vi "__Destroy.vi"(8 "error in (no error)":errorcluster, 11 "ClashRoyale in":refnum<class "ClashRoyale.lvclass">) -> (0 "error out":errorcluster)   [LabVIEW 2020, in "ClashRoyale.lvclass"]
uses:
  ClashRoyale.lvclass
  ClashRoyale.lvclass/ClashRoyale.ctl
  <vilib>/drjdpowell/SQLite Library/SQL Connection/Connection.lvclass
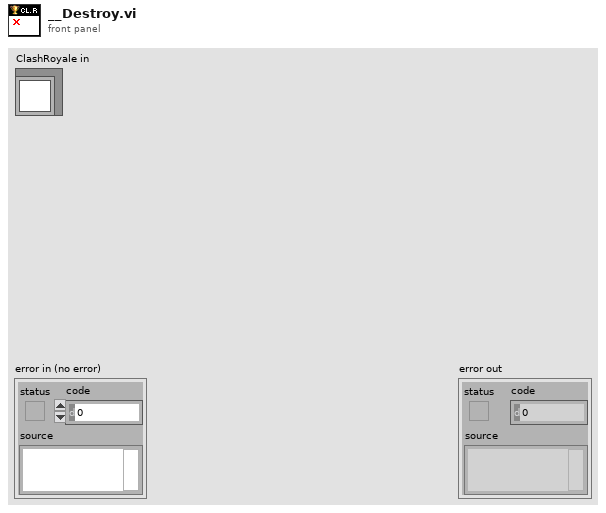
[diagram p1: front panel]
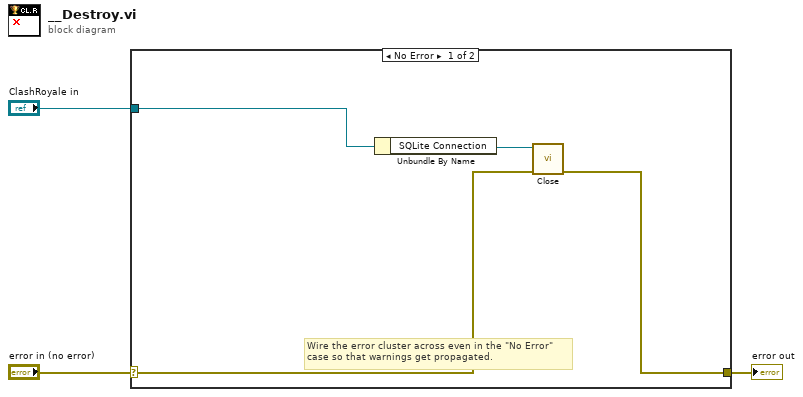
[diagram p0: block diagram]
diagram:
  n1 = case shown="No Error" "error in (no error)" {
    selector: "error in (no error)" -> [w7 w8]
    tunnel: [w6 w8] -> w2
    tunnel: "ClashRoyale in" -> [w5 _]
    frame No Error {
      # "Wire the error cluster across even in the \"No Error\"\ncase so that warnings get propagated."
      n2 = Unbundle By Name(w5) -> ("SQLite Connection"=w4:refnum<class "Connection.lvclass">)
      n3 = call-dynamic "Close.vi"("error in (no error)"=w7, "SQLite Connection in"=w4) -> ("error out"=w6:errorcluster)  [unwired: 9 in]
    }
    frame Error {
    }
  }
  "error out" <- w2
